vi "write_pdo_mapping.vi"(9 "data":u32, 10 "subind":u8, 11 "index":u16) -> (3 "return":i16)   [LabVIEW 2011]
uses:
  canopen_dll_master.dll
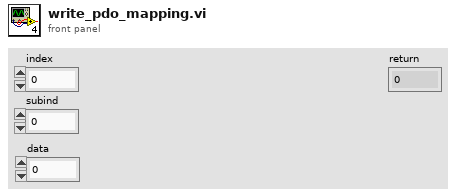
[diagram p1: front panel]
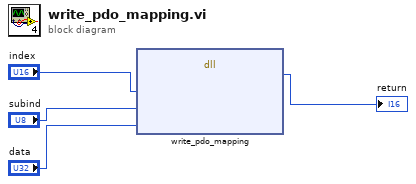
[diagram p0: block diagram]
diagram:
  n1 = dll-call lib="canopen_dll_master.dll" fn="write_pdo_mapping"("index"="index", "subind"="subind", "data"="data") -> ("return type"=→"return":i16)  [unwired: 6 in, 2 out]
